vi "Read Test Case Results.vi"(11 "Test Suite Result In":refnum<class "Test Suite Result.lvclass">) -> (2 "Case Results":refnum<class "Test Case Result.lvclass">[](array[class]), 3 "Test Suite Result Out":refnum<class "Test Suite Result.lvclass">)   [LabVIEW 2020, in "Test Suite Result.lvclass"]
uses:
  Test Suite Result.lvclass
  Test Case Result/Test Case Result.lvclass
  Test Suite Result.lvclass/Test Suite Result.ctl
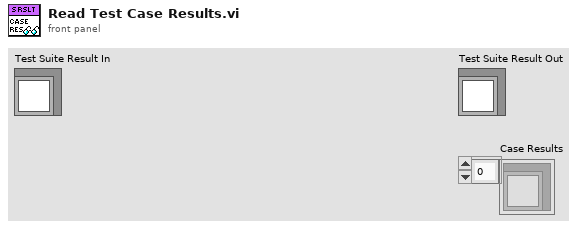
[diagram p1: front panel]
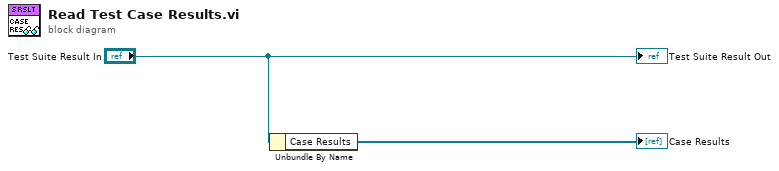
[diagram p0: block diagram]
diagram:
  n1 = Unbundle By Name("Test Suite Result In") -> ("Case Results"=→"Case Results":refnum<class "Test Case Result.lvclass">[])
  "Test Suite Result Out" <- "Test Suite Result In"
